vi "Rd Wr detector settings json.vi"(7 "Detector Name":string="Default", 8 "error in (no error)":errorcluster, 9 "Settings File":string="CC System Settings.json", 10 "Write? (F:Read)":bool, 11 "Detector Config":T4={"Detector"=0, "Offsets"=[[0, 0, 0, 0, 0, 0, 0, 0, 0, 0, 0, 0, 0, 0, 0, 0, 0, 0, 0, 0, 0, 0, 0, 0, 0, 0, 0, 0, 0, 0, 0, 0]], "Detector Computer"={"Machine"="192.168.121.11", "Password"="R!MAS1grb", "FITS File Path"="/local/data/fermi-grb1/home/rimas/dev/h2rg/fitdat", "Port"=44444, "Header Path"="/local/data/fermi-grb1/home/rimas/dev/h2rg/header", "Name"="Simulation"}, "FITS hdr template0"=path "C:/Users/gsfcprime/Documents/LabVIEW Data/FITS Templates/header0.dat", "FITS hdr template1"=path "C:/Users/gsfcprime/Documents/LabVIEW Data/FITS Templates/header1.dat", "FITS Data File Path"=path "C:/Users/gsfcprime/Documents/LabVIEW Data/PRIME FITS Images", "FITS Detector Settings"={"Exp Time Short"=1.0, "# of Frames"=1.0, "Exp Time Long"=2.0, "# of Groups"=1.0, "Object Name"="", "Object"="", "Obs Type"="", "Image Type"="", "Observer"="", "Observer Affiliation"=""}, "Sim Folder"=path "C:/Users/gsfcprime/Documents/LabVIEW Data/PRIME Simulation FITS Images", "Integration Mode"=enum."SSR", "Integration Time"=0.0, "Frame Int Time"=0.0} {"Offsets" format="%04x"; "Detector" items=["0", "1", "2"]}) -> (0 "error out":errorcluster, 3 "Detector Config":T4={"Detector"=0, "Offsets"=[[0, 0, 0, 0, 0, 0, 0, 0, 0, 0, 0, 0, 0, 0, 0, 0, 0, 0, 0, 0, 0, 0, 0, 0, 0, 0, 0, 0, 0, 0, 0, 0]], "Detector Computer"={"Machine"="192.168.121.11", "Password"="", "FITS File Path"="", "Port"=44444, "Header Path"="", "Name"=""}, "FITS hdr template0"=path "", "FITS hdr template1"=path "", "FITS Data File Path"=path "", "FITS Detector Settings"={"Exp Time Short"=0.0, "# of Frames"=0.0, "Exp Time Long"=0.0, "# of Groups"=0.0, "Object Name"="", "Object"="", "Obs Type"="", "Image Type"="", "Observer"="", "Observer Affiliation"=""}, "Sim Folder"=path "", "Integration Mode"=enum."SSR", "Integration Time"=0.0, "Frame Int Time"=0.0} {"Offsets" format="%04x"; "Detector" items=["0", "1", "2"]})   [LabVIEW 2021]
uses:
  RIMAS Detector Config.ctl
  RIMAS Detector Server Config.ctl
  RIMAS Observation Config.ctl
  Detector Class/Detector enum Detector Integration Mode.ctl
  2e80df6d-94aa-46b9-8b94-ceea8c057880.vi
  659fb017-0e9f-42f9-b06e-930303f00cbc.vi
  <vilib>/JDP Science/JSONtext/Find Item.vi
  <vilib>/JDP Science/JSONtext/Next JSON Value.vi
  <vilib>/JDP Science/JSONtext/String Subset.vi
  <vilib>/JDP Science/JSONtext/Parsing/Advance past next JSON Value (inlined COPY).vi
  <vilib>/JDP Science/JSONtext/Parsing/Advance past whitespace.vi
  <vilib>/JDP Science/JSONtext/Parsing/Advance past String.vi
  <vilib>/JDP Science/JSONtext/Parsing/Advance past Number.vi
  <vilib>/JDP Science/JSONtext/Parsing/Advance past Line Ending.vi
  <vilib>/JDP Science/JSONtext/Parsing/Parse Full Path or Item Name.vi
  <vilib>/JDP Science/JSONtext/Parsing/Advance past Array.vi
  <vilib>/JDP Science/JSONtext/Parsing/Advance past Object.vi
  <vilib>/JDP Science/JSONtext/support/Error Cluster From Code.vi
  <vilib>/JDP Science/JSONtext/Offset/Find Item Locations by Path.vi
  <vilib>/JDP Science/JSONtext/JSON text to Variant.vi
  <vilib>/JDP Science/JSONtext/Variant to JSON Text.vi
  <vilib>/JDP Science/JSONtext/Set Item.vi
  <vilib>/JDP Science/JSONtext/LVClass Serializer/JSONtext LVClass Serializer.lvclass
panel:
  in  "Detector Config 2":T3={"Detector"=0, "Offsets 0"=[0, 0, 0, 0, 0, 0, 0, 0, 0, 0, 0, 0, 0, 0, 0, 0, 0, 0, 0, 0, 0, 0, 0, 0, 0, 0, 0, 0, 0, 0, 0, 0], "Detector Computer"={"Machine"="192.168.121.11", "Password"="R!MAS1grb", "FITS File Path"="/local/data/fermi-grb1/home/rimas/dev/h2rg/fitdat", "Port"=44444, "Header Path"="/local/data/fermi-grb1/home/rimas/dev/h2rg/header", "Name"="Simulation"}, "FITS hdr template0"=path "C:/Users/gsfcprime/Documents/LabVIEW Data/FITS Templates/header0.dat", "FITS hdr template1"=path "C:/Users/gsfcprime/Documents/LabVIEW Data/FITS Templates/header1.dat", "FITS Data File Path"=path "C:/Users/gsfcprime/Documents/LabVIEW Data/PRIME FITS Images", "FITS Detector Settings"={"Exp Time Short"=1.0, "# of Frames"=1.0, "Exp Time Long"=2.0, "# of Groups"=1.0, "Object Name"="", "Object"="", "Obs Type"="", "Image Type"="", "Observer"="", "Observer Affiliation"=""}, "Offsets 1"=[0, 0, 0, 0, 0, 0, 0, 0, 0, 0, 0, 0, 0, 0, 0, 0, 0, 0, 0, 0, 0, 0, 0, 0, 0, 0, 0, 0, 0, 0, 0, 0], "Sim Folder"=path "C:/Users/gsfcprime/Documents/LabVIEW Data/PRIME Simulation FITS Images"} {"Offsets 1" format="%04x"; "Offsets 0" format="%04x"; "Detector" items=["0", "1", "2"]}
  # "sec"
  # "sec"
  # "sec"
  # "sec"
  # "sec"
  # "sec"
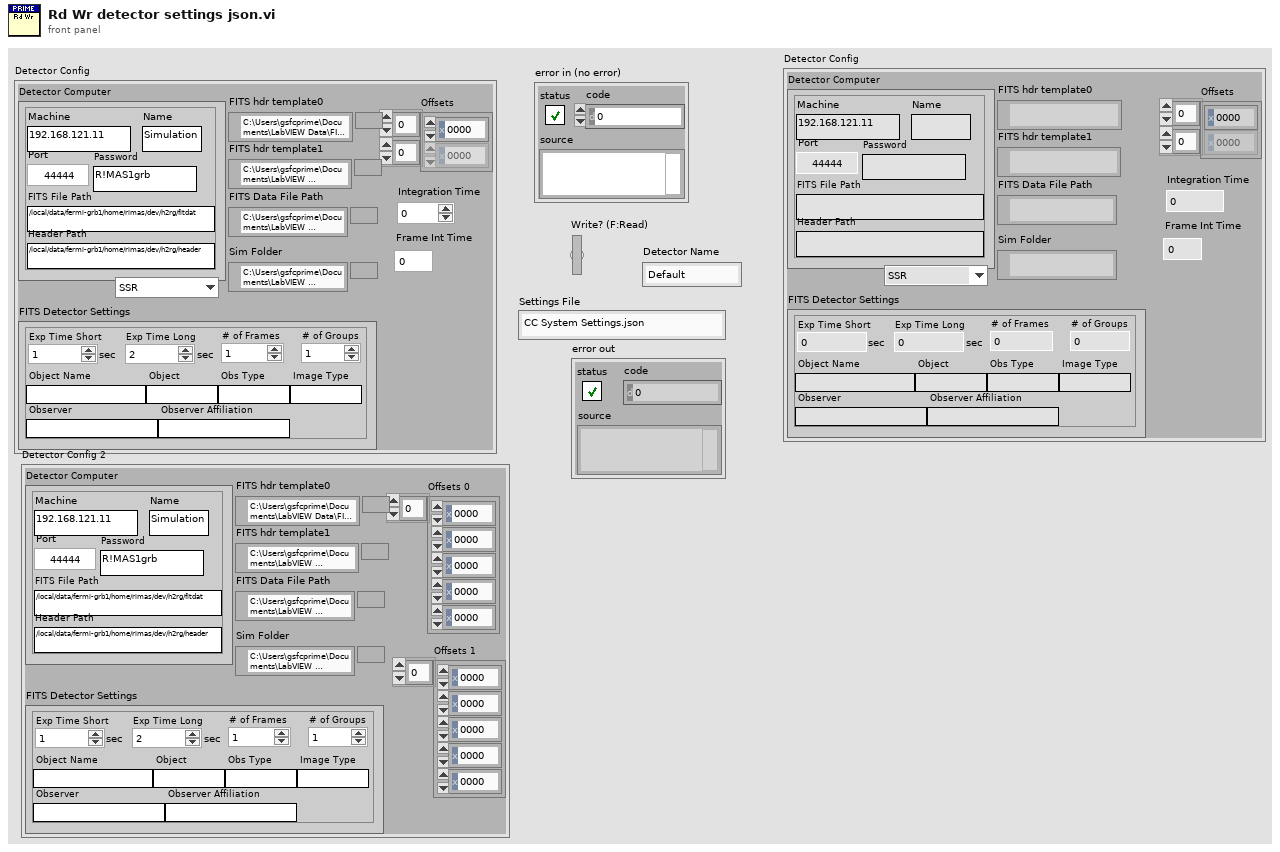
[diagram p1: front panel]
types:
  T1 = typedef "RIMAS Detector Server Config.ctl" = cluster{"Machine":string, "Password":string, "FITS File Path":string, "Port":u16, "Header Path":string, "Name":string}
  T2 = typedef "RIMAS Observation Config.ctl" = cluster{"Exp Time Short":dbl, "# of Frames":dbl, "Exp Time Long":dbl, "# of Groups":dbl, "Object Name":string, "Object":string, "Obs Type":string, "Image Type":string, "Observer":string, "Observer Affiliation":string}
  T3 = cluster{"Detector":u16, "Offsets 0":u16[], "Detector Computer":T1, "FITS hdr template0":path, "FITS hdr template1":path, "FITS Data File Path":path, "FITS Detector Settings":T2, "Offsets 1":u16[], "Sim Folder":path}
  T4 = typedef "RIMAS Detector Config.ctl" = cluster{"Detector":u16, "Offsets":u16[][], "Detector Computer":T1, "FITS hdr template0":path, "FITS hdr template1":path, "FITS Data File Path":path, "FITS Detector Settings":T2, "Sim Folder":path, "Integration Mode":T5, "Integration Time":dbl, "Frame Int Time":dbl}
  T5 = typedef "Detector enum Detector Integration Mode.ctl" = enum16{"SSR", "CDS", "MEAN", "MEDIAN", "MODE", "MIIN", "MAX"}
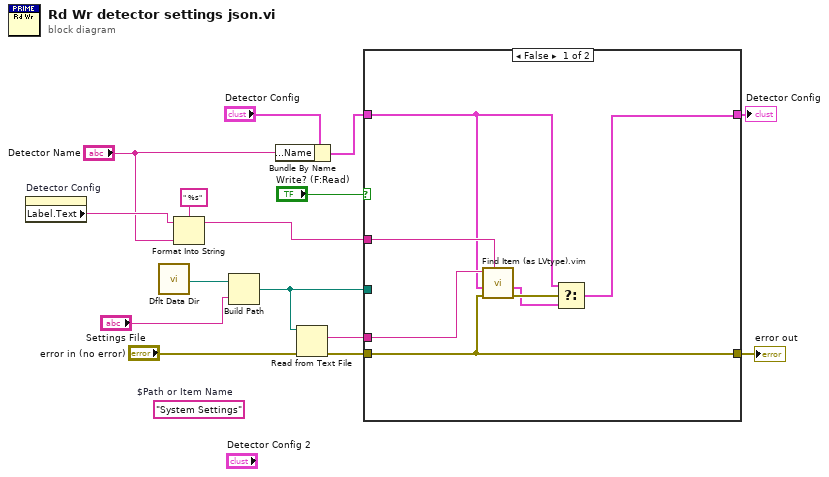
[diagram p0: block diagram]
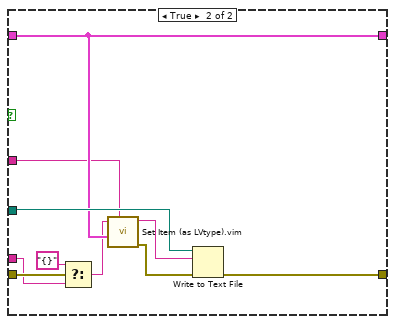
[diagram p2: hidden frame]
diagram:
  (unwired) "System Settings"  # $Path or Item Name
  n1 = property on="Detector Config" class="Clust (strict)"() -> ("Label.Text"=w5:string)  [unwired: 2 in, 2 out]
  n2 = call <vilib>:"Dflt Data Dir.vi"() -> ("App:Default Data Directory"=w13:path)
  n3 = Format Into String(format string=" %s", initial string=w5, "Detector Name") -> (resulting string=w4:string)  [unwired: 1 in, 1 out]
  n4 = Build Path(base path=w13, name or relative path="Settings File") -> (appended path=w7:path)
  n5 = Bundle By Name(cluster="Detector Config", "Detector Computer.Name"="Detector Name") -> (w1:T4)
  n6 = Read from Text File(file (use dialog)=w7, error in="error in (no error)") -> (text=w8:string, error out=w9:errorcluster)  [unwired: 2 in, 2 out]
  n7 = case shown="False" "Write? (F:Read)" {
    tunnel: w9 -> [w17 w27]
    tunnel: w1 -> [w16 w30]
    tunnel: w7 -> [_ w32]
    tunnel: [w17 w31] -> w12
    tunnel: [w22 w30] -> w11
    tunnel: w4 -> [w21 w29]
    tunnel: w8 -> [w18 w25]
    frame False {
      n8 = call "Find Item (as LVtype).vim"("$Path or Item Name"=w21, "error in (no error)"=w17, "Data Type and Default Value"=w16, "JSON"=w18) -> ("error out"=w20:errorcluster, "Data"=w19:T4)  [unwired: 4 in, 2 out]
      n9 = Select(t=w16, s=w20, f=w19) -> (s? t:f=w22:T4)
    }
    frame True {
      n10 = Select(t="{}" ("JSON"), s=w27, f=w25) -> (s? t:f=w24:string)
      n11 = call "Set Item (as LVtype).vim"("$Path or Item Name"=w29, "Anything"=w30, "JSON"=w24) -> ("error out"=w23:errorcluster, "<JSON>"=w28:string)  [unwired: 5 in, 1 out]
      n12 = Write to Text File(file (use dialog)=w32, text=w28, error in=w23) -> (error out=w31:errorcluster)  [unwired: 1 in, 2 out]
    }
  }
  "error out" <- w12
  "Detector Config" <- w11
